vi "StageInit.vi"(8 "error in (no error)":errorcluster, 11 "StageHandle In":T3) -> (0 "error out":errorcluster, 2 "Device Out":T1, 3 "StageHandle Out":T2)   [LabVIEW 2014]
doc: "This is used to initialize the 3 traslation stages"
uses:
  C:/Users/light/Desktop/SI+Raman/Labview/Raman/dll/Thorlabs.MotionControl.Controls.dll
  dll/Thorlabs.MotionControl.Controls.dll
  C:/Users/light/Desktop/SI+Raman/Labview/Raman/dll/ThorLabs.MotionControl.KCube.DCServoCLI.dll
  dll/ThorLabs.MotionControl.KCube.DCServoCLI.dll
  TypeDef/StageDeviceOut.ctl
  TypeDef/StageHandleIn.ctl
  TypeDef/StageHandleOut.ctl
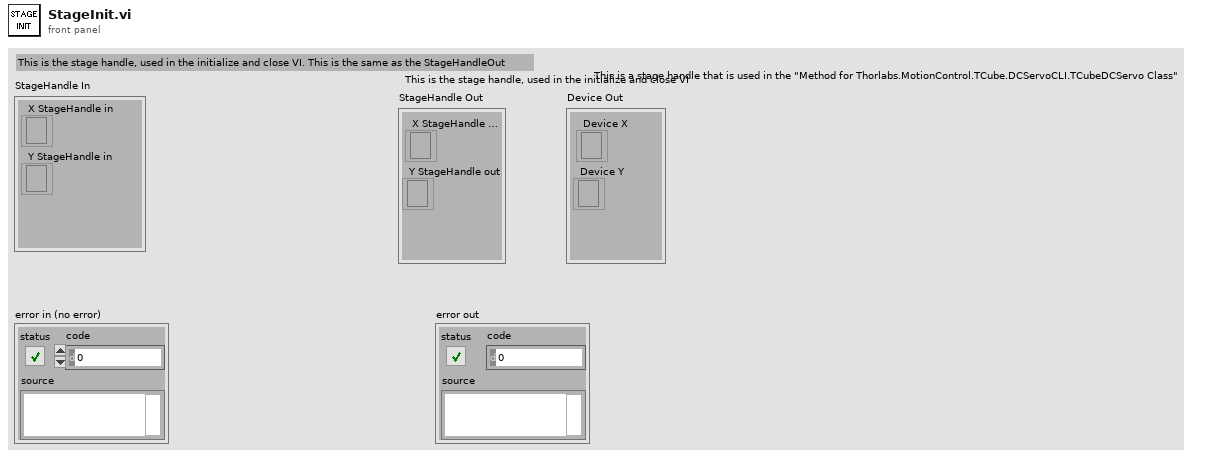
[diagram p1: front panel]
types:
  T1 = typedef "StageDeviceOut.ctl" = cluster{"Device X":refnum<k24>, "Device Y":refnum<k24>}
  T2 = typedef "StageHandleOut.ctl" = cluster{"X StageHandle out":refnum<k24>, "Y StageHandle out":refnum<k24>}
  T3 = typedef "StageHandleIn.ctl" = cluster{"X StageHandle in":refnum<k24>, "Y StageHandle in":refnum<k24>}
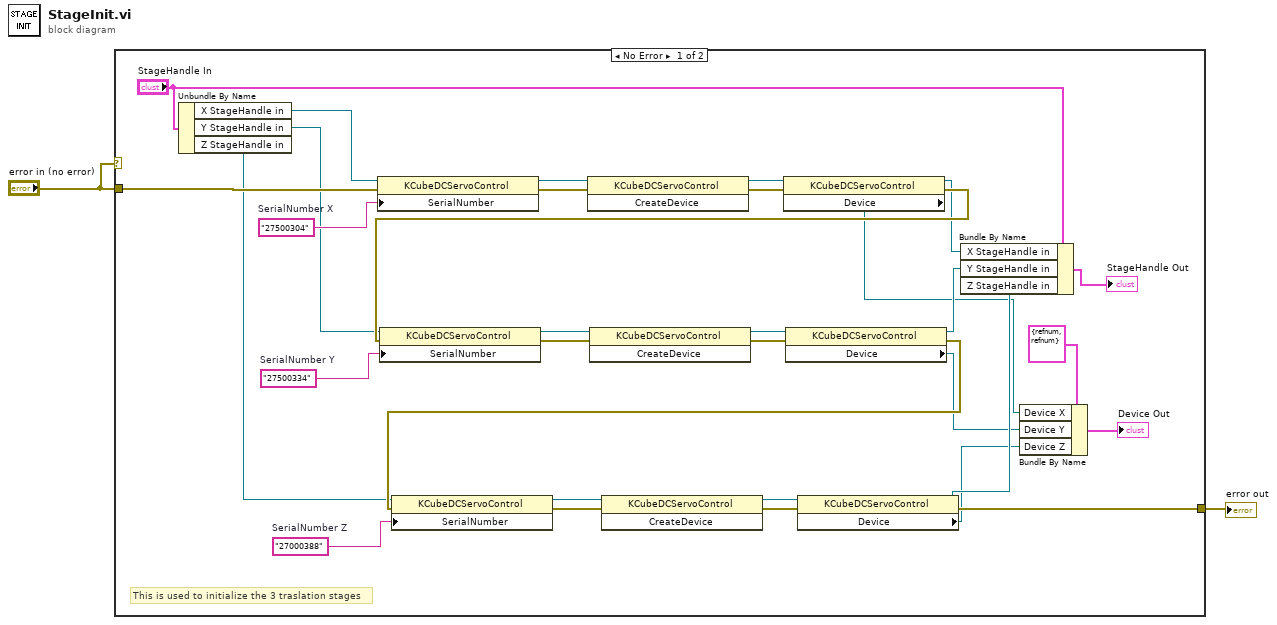
[diagram p0: block diagram]
diagram:
  n1 = case shown="No Error" "error in (no error)" {
    tunnel: [w29 w35] -> w2
    tunnel: "error in (no error)" -> [w18 w35]
    frame No Error {
      w23 = "27500334"  # SerialNumber Y
      w28 = "27500304"  # SerialNumber X
      w34 = "27000388"  # SerialNumber Z
      # "This is used to initialize the 3 traslation stages"
      n2 = Unbundle By Name("StageHandle In") -> ("X StageHandle in"=w15:refnum<k24>, "Y StageHandle in"=w14:refnum<k24>, "Z StageHandle in"=w13:refnum<k24>)
      n3 = property class="KCubeDCServoControl"(reference=w15, error in=w18, "SerialNumber"=w28) -> (reference out=w27:refnum<k24>, error out=w26:errorcluster)
      n4 = invoke class="KCubeDCServoControl" method="CreateDevice"(reference=w27, error in=w26) -> (reference out=w25:refnum<k24>, error out=w24:errorcluster)  [unwired: 1 in, 1 out]
      n5 = property class="KCubeDCServoControl"(reference=w25, error in=w24) -> (reference out=w11:refnum<k24>, error out=w17:errorcluster, "Device"=w5:refnum<k24>)
      n6 = property class="KCubeDCServoControl"(reference=w14, error in=w17, "SerialNumber"=w23) -> (reference out=w22:refnum<k24>, error out=w21:errorcluster)
      n7 = invoke class="KCubeDCServoControl" method="CreateDevice"(reference=w22, error in=w21) -> (reference out=w20:refnum<k24>, error out=w19:errorcluster)  [unwired: 1 in, 1 out]
      n8 = property class="KCubeDCServoControl"(reference=w20, error in=w19) -> (reference out=w10:refnum<k24>, error out=w16:errorcluster, "Device"=w4:refnum<k24>)
      n9 = property class="KCubeDCServoControl"(reference=w13, error in=w16, "SerialNumber"=w34) -> (reference out=w33:refnum<k24>, error out=w32:errorcluster)
      n10 = invoke class="KCubeDCServoControl" method="CreateDevice"(reference=w33, error in=w32) -> (reference out=w31:refnum<k24>, error out=w30:errorcluster)  [unwired: 1 in, 1 out]
      n11 = property class="KCubeDCServoControl"(reference=w31, error in=w30) -> (reference out=w9:refnum<k24>, error out=w29:errorcluster, "Device"=w3:refnum<k24>)
      n12 = Bundle By Name(cluster="StageHandle In", "X StageHandle in"=w11, "Y StageHandle in"=w10, "Z StageHandle in"=w9) -> (→"StageHandle Out":T3)
      n13 = Bundle By Name(cluster=T1 {"Device X"=refnum, "Device Y"=refnum} ("Device Out 2"), "Device X"=w5, "Device Y"=w4, "Device Z"=w3) -> (→"Device Out":T1)
    }
    frame Error {
    }
  }
  "error out" <- w2
